vi "Receive.vi"(10 "Msg Strategy in":refnum<class "Msg Strategy.lvclass">, 11 "TEMPLATE Event in":refnum<class "TEMPLATE Event.lvclass">) -> (2 "Msg Strategy out":refnum<class "Msg Strategy.lvclass">, 3 "TEMPLATE Event out":refnum<class "TEMPLATE Event.lvclass">)   [LabVIEW 2021, in "_Template.lvlib" / "Templates.lvlib" / "TEMPLATE Event.lvlib" / "TEMPLATE Event.lvclass"]
uses:
  TEMPLATE Event.lvclass
  TEMPLATE Event.lvclass/TEMPLATE Event.ctl
  jettl/jettl/Event/Event.lvclass
  jettl/jettl/Msg Strategy/Msg Strategy.lvclass
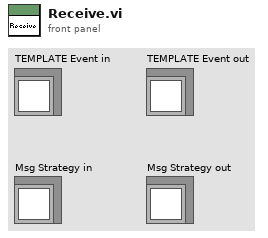
[diagram p1: front panel]
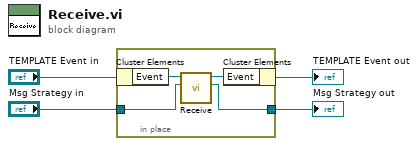
[diagram p0: block diagram]
diagram:
  n1 = in-place {
    in-place-border: "Msg Strategy in" -> [w7]
    in-place-border: [w6] -> w1
    n2 = in-place-cluster #1("TEMPLATE Event in") -> ("Event"=w8:refnum<class "Event.lvclass">)
    n3 = call-dynamic "Receive.vi"("Msg Strategy in"=w7, "Event in"=w8) -> ("Msg Strategy out"=w6:refnum<class "Msg Strategy.lvclass">, "Event out"=w5:refnum<class "Event.lvclass">)  [unwired: 8 in]
    n4 = in-place-cluster #1("Event"=w5) -> (→"TEMPLATE Event out":refnum<class "TEMPLATE Event.lvclass">)
  }
  "Msg Strategy out" <- w1
